vi "Read Next Message.vi"(7 "States In":string, 8 "Error in (no error)":errorcluster, 9 "timeout (1ms)":i32, 11 "Message Queue in":T1) -> (0 "Error out":errorcluster, 1 "Arguments":string, 2 "Current State":string, 3 "Message Queue out":T1, 4 "Exit Process":bool, 5 "Remaining States":string, 6 "Current State With Arguments":string)   [LabVIEW 2017]
uses:
  subVIs/TypeDefs/amc_Message Queue.ctl
  subVIs/TypeDefs/amc_Message.ctl
  Tools/Keyed Array/Tools_KeyedArray KeyedArray.ctl
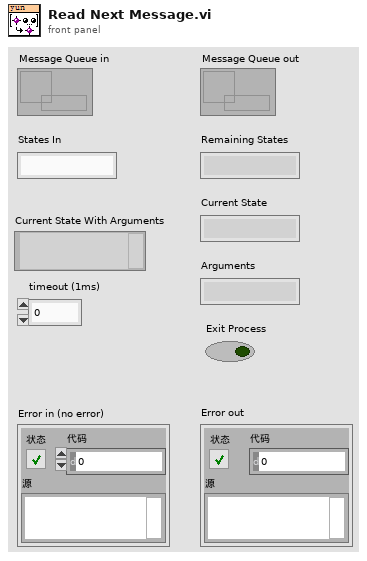
[diagram p1: front panel]
types:
  T1 = typedef "amc_Message Queue.ctl" = refnum<queue>
  T2 = typedef "amc_Message.ctl" = cluster{"Name":string, "Value":string, "Attributes":T3, "Receiver Host":string, "Receiver Process":string, "Source Host":string, "Source Process":string, "Priority Message":bool, "Acknowledge Message":bool}
  T3 = typedef "Tools_KeyedArray KeyedArray.ctl" = cluster{"keys":string[], "values":string[]}
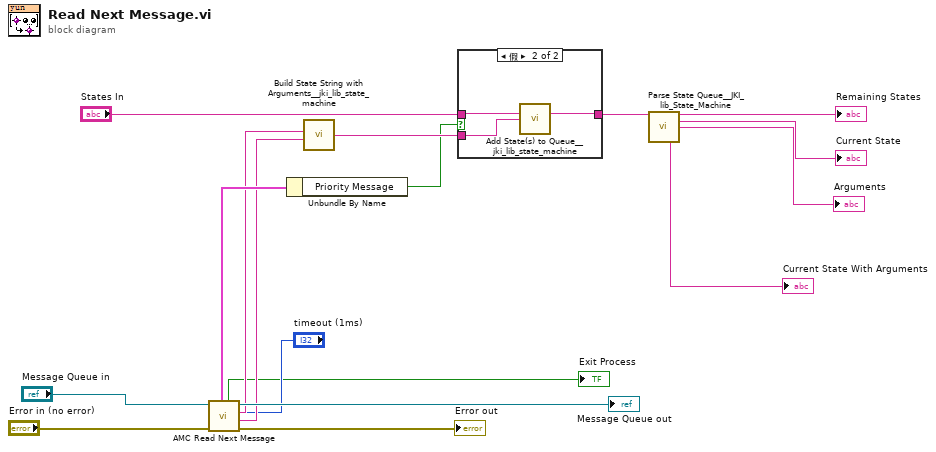
[diagram p0: block diagram]
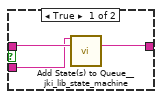
[diagram p2: hidden frame]
diagram:
  n1 = call "AMC Read Next Message.vi"("error in (no error)"="Error in (no error)", "timeout (1ms)"="timeout (1ms)", "Message Queue in"="Message Queue in") -> ("error out"=→"Error out":errorcluster, "Message Value"=w10:string, "Message Name"=w9:string, "Message Queue out"=→"Message Queue out":T1, "Exit Process"=→"Exit Process":bool, "Message"=w15:T2)  [unwired: 1 in, 2 out]
  n2 = Unbundle By Name(w15) -> ("Priority Message"=w16:bool)
  n3 = call "Build State String with Arguments__jki_lib_state_machine.vi"("Arguments (\"\")"=w10, "State"=w9) -> ("State with Arguments"=w17:string)  [unwired: 4 in]
  n4 = case shown="假" w16 {
    tunnel: "States In" -> [w20 w23]
    tunnel: [w19 w22] -> w8
    tunnel: w17 -> [w18 w21]
    frame True {
      n5 = call "Add State(s) to Queue__jki_lib_state_machine.vi"("State(s) in Front (\"\")"=w18, "State(s) in (\"\")"=w20) -> ("States Out"=w19:string)  [unwired: 13 in]
    }
    frame False {
      n6 = call "Add State(s) to Queue__jki_lib_state_machine.vi"("State(s) in (\"\")"=w23, "State(s) at Back (\"\")"=w21) -> ("States Out"=w22:string)  [unwired: 13 in]
    }
  }
  n7 = call "Parse State Queue__JKI_lib_State_Machine.vi"("State Queue"=w8) -> ("Remaining States"=→"Remaining States":string, "Current State"=→"Current State":string, "Arguments"=→"Arguments":string, "Current State With Arguments"=→"Current State With Arguments":string)  [unwired: 11 in]
